vi "Write DER SetpointV.vi"(8 "error in":errorcluster, 10 "DER_SetPointV":T1, 11 "DER in":refnum<class "DER.lvclass">) -> (0 "error out":errorcluster, 3 "DER out":refnum<class "DER.lvclass">)   [LabVIEW 2018, in "DER Actor.lvlib" / "DER.lvclass"]
uses:
  DER.lvclass
  C:/Users/Administrator/Desktop/2018LabVIEW EMS/IED Actors/Device DDS Communications Framework/Device DDS Communications/Device DDS Communications.lvclass
  <vilib>/ORNL/CSEISMIC DDS/CSEISMIC DDS Base/Data Types/DER_SetPointV.ctl
  <vilib>/ORNL/CSEISMIC DDS/CSEISMIC DDS Base/Data Types/Controls/DeviceID.ctl
  Device DDS Communications Framework/Device DDS Communications/Device DDS Communications.lvclass/Device DDS Communications.ctl
  <vilib>/ORNL/CSEISMIC DDS/CSEISMIC DDS Base/CSEISMIC DDS.lvclass/CSEISMIC DDS.ctl
  <vilib>/ORNL/CSEISMIC DDS/CSEISMIC DDS Base/Accessors/Read DDS Reference.vi
  <vilib>/ORNL/CSEISMIC DDS/DDS Writer/DDS Writer.lvclass
  C:/Program Files (x86)/National Instruments/LabVIEW 2018/vi.lib/ORNL/CSEISMIC DDS/CSEISMIC DDS Base/CSEISMIC DDS.lvclass
  <vilib>/ORNL/CSEISMIC DDS/CSEISMIC DDS Base/Error Handler.vi
  Device DDS Communications Framework/Device DDS Communications/Device DDS Communications.lvclass
  <vilib>/ORNL/CSEISMIC DDS/CSEISMIC DDS Base/CSEISMIC DDS.lvclass
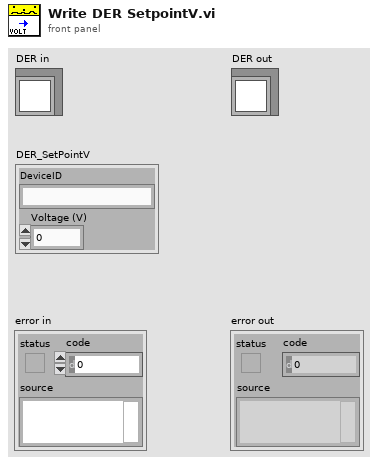
[diagram p1: front panel]
types:
  T1 = typedef "CSEISMIC DDS.lvlib/CSEISMIC DDS.lvclass/DER_SetPointV.ctl" = cluster{"DeviceID":T2, "Voltage (V)":dbl}
  T2 = typedef "CSEISMIC DDS.lvlib/CSEISMIC DDS.lvclass/DeviceID.ctl" = string
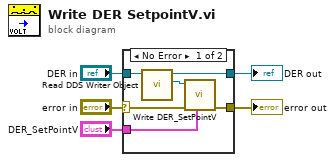
[diagram p0: block diagram]
diagram:
  n1 = case shown="No Error" "error in" {
    selector: "error in" -> [w8 w13]
    tunnel: [w7 w13] -> w4
    tunnel: [w10 w12] -> w2
    tunnel: "DER in" -> [w11 w12]
    tunnel: "DER_SetPointV" -> [w6 _]
    frame No Error {
      n2 = call "Read DDS Writer Object.vi"("Device DDS Communications in"=w11) -> ("DDS Writer Object"=w9:refnum<class "DDS Writer.lvclass">, "Device DDS Communications out"=w10:refnum<class "DER.lvclass">)  [unwired: 9 in]
      n3 = call <vilib>:"Write DER_SetPointV.vi"("DER_SetPointV"=w6, "error in"=w8, "DDS Writer in"=w9) -> ("error out"=w7:errorcluster)  [unwired: 7 in, 1 out]
    }
    frame Error {
    }
  }
  "error out" <- w4
  "DER out" <- w2
